vi "Create Circle Single.vi"(9 "M Point":dbl[](array[numeric]), 10 "Points N":i32, 11 "Radius":dbl) -> (2 "Y":dbl[](array[numeric]), 3 "X":dbl[](array[numeric]))   [LabVIEW 2020, in "Settings.lvlib"]
uses:
  Settings.lvlib
  <vilib>/Analysis/NI_AALBase.lvlib
panel:
  out "Waveform Graph":dbl[][](graph)
  out "XY Graph":cluster{"X":dbl[], "Y":dbl[]}[](graph)
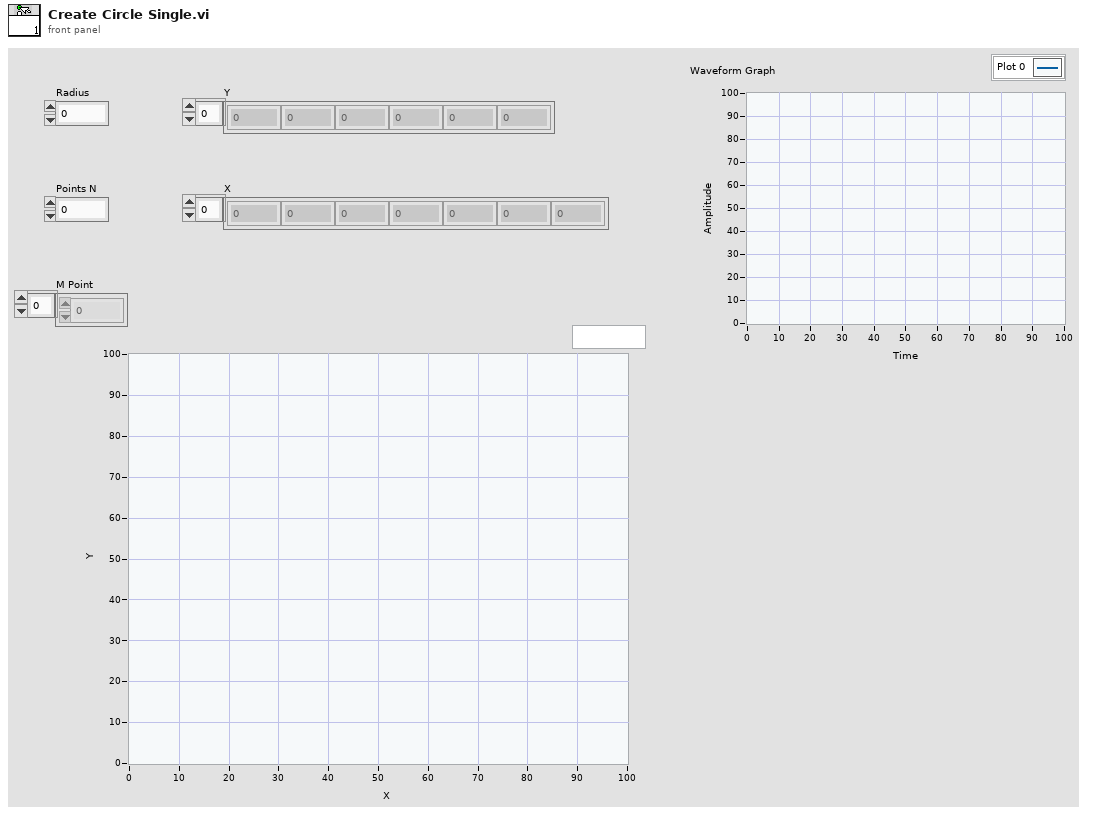
[diagram p1: front panel]
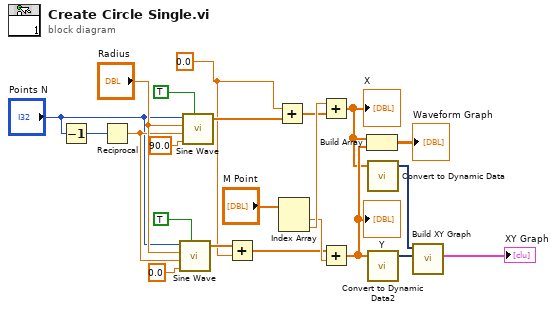
[diagram p0: block diagram]
diagram:
  w1 = 0.0 ("phase in")
  n1 = Decrement(x="Points N") -> (x-1=w4:i32)
  n2 = Reciprocal(x=w4) -> (1/x=w18:dbl)
  n3 = call <vilib>:"Sine Wave.vi"("samples"="Points N", "amplitude"="Radius", "frequency"=w18, "phase in"=0.0, "reset phase"=TRUE) -> ("sine wave"=w12:dbl[])  [unwired: 2 out]
  n4 = call <vilib>:"Sine Wave.vi"("samples"="Points N", "amplitude"="Radius", "frequency"=w18, "phase in"=90.0, "reset phase"=TRUE) -> ("sine wave"=w13:dbl[])  [unwired: 2 out]
  n5 = Add(x=w12, y=w1) -> (x+y=w14:dbl[])
  n6 = Add(x=w1, y=w13) -> (x+y=w15:dbl[])
  n7 = Index Array(array="M Point") -> (element #1=w21:dbl, element #2=w22:dbl)  [unwired: 2 in]
  n8 = Add(x=w22, y=w15) -> (x+y=w2:dbl[])
  "X" <- w2
  n9 = Add(x=w14, y=w21) -> (x+y=w3:dbl[])
  "Y" <- w3
  n10 = Build Array(w2, w3) -> (→"Waveform Graph":dbl[][])
  n11 = call "Convert to Dynamic Data"("Array"=w2) -> ("Dynamic Data Type"=w9:dynamicdata)  [unwired: 3 in]
  n12 = call "Convert to Dynamic Data2"("Array"=w3) -> ("Dynamic Data Type"=w8:dynamicdata)  [unwired: 3 in]
  n13 = call "Build XY Graph"("Y Input"=w8, "X Input"=w9) -> ("XY Graph"=→"XY Graph":cluster{"X":dbl[], "Y":dbl[]}[])  [unwired: 8 in, 1 out]
